vi "Aeroflex8311_SetAttenuation.vi"(1 "error in (no error)":errorcluster, 2 "Attenuation (dB)":dbl, 3 "Channel":dbl, 4 "VISA resource name":refnum<visa-resource-name>="GPIB0::10::INSTR") -> (0 "error out":T1)   [LabVIEW 2014]
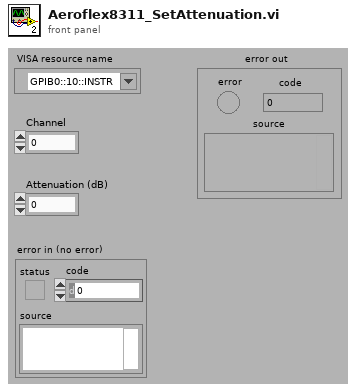
[diagram p1: front panel]
types:
  T1 = cluster{"error":bool, "code":i32, "source":string}
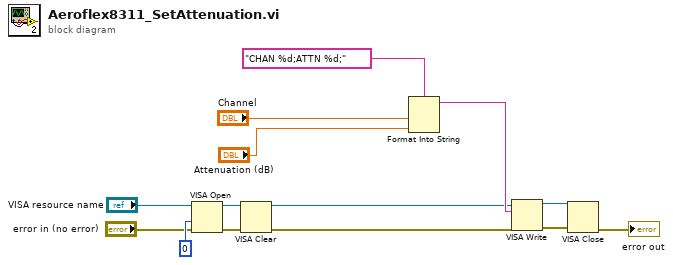
[diagram p0: block diagram]
diagram:
  n1 = VISA Open(access mode=u32 0, error in (no error)="error in (no error)", VISA resource name="VISA resource name") -> (VISA resource name=w10:refnum<visa-resource-name>, error out=w9:errorcluster)  [unwired: 2 out]
  n2 = VISA Clear(VISA resource name=w10, error in (no error)=w9) -> (VISA resource name out=w6:refnum<visa-resource-name>, error out=w5:errorcluster)
  n3 = Format Into String(format string="CHAN %d;ATTN %d;", "Channel", "Attenuation (dB)") -> (resulting string=w14:string)  [unwired: 2 in, 1 out]
  n4 = VISA Write(VISA resource name=w6, write buffer=w14, error in (no error)=w5) -> (VISA resource name out=w4:refnum<visa-resource-name>, error out=w3:errorcluster)  [unwired: 1 out]
  n5 = VISA Close(VISA resource name=w4, error in (no error)=w3) -> (error out=→"error out":errorcluster)
